vi "03122013A.vi"() -> ()   [LabVIEW 2012]
panel:
  out "Y min":dbl format="%0.2f"
  out "Y max":dbl format="%0.2f"
  in  "dt":dbl
  out "Waveform Chart 2":waveform(dbl)(graph)
  out "output waveform":waveform(dbl)
  out "XY Graph":cluster{"Y":dbl[], "Y":dbl[]}[](graph)
  out "Waveform Graph":cluster{"Xo":i32, "dx":i32, dbl[]}(graph)
  in  "Scale Legend:Visible":bool
  in  "Data on Demand":bool
  in  "X Scale.Style":u8
  out "File Status":bool
  out "Elapsed Time Text":string
  out "Waveform Chart":cluster{i32, "Elapsed Time (s)":dbl, dbl}(graph)
  in  "access (0:read/write)":enum16{"read/write", "read-only", "write-only"}(ring)
  out "output cluster":cluster{string, string, string}
  in  "operation (0:open) 2":T1(ring)
  in  "file path (use dialog) 2":path
  in  "Scan Control":dbl(knob)=250.0 scale=0.0..5000.0
  out "Data Panel":T2 {"Elapsed Time (s)" format="%#_5f"}
  out "error out":errorcluster
  out "Array":dbl[][](array[numeric])
  in  "stop":bool
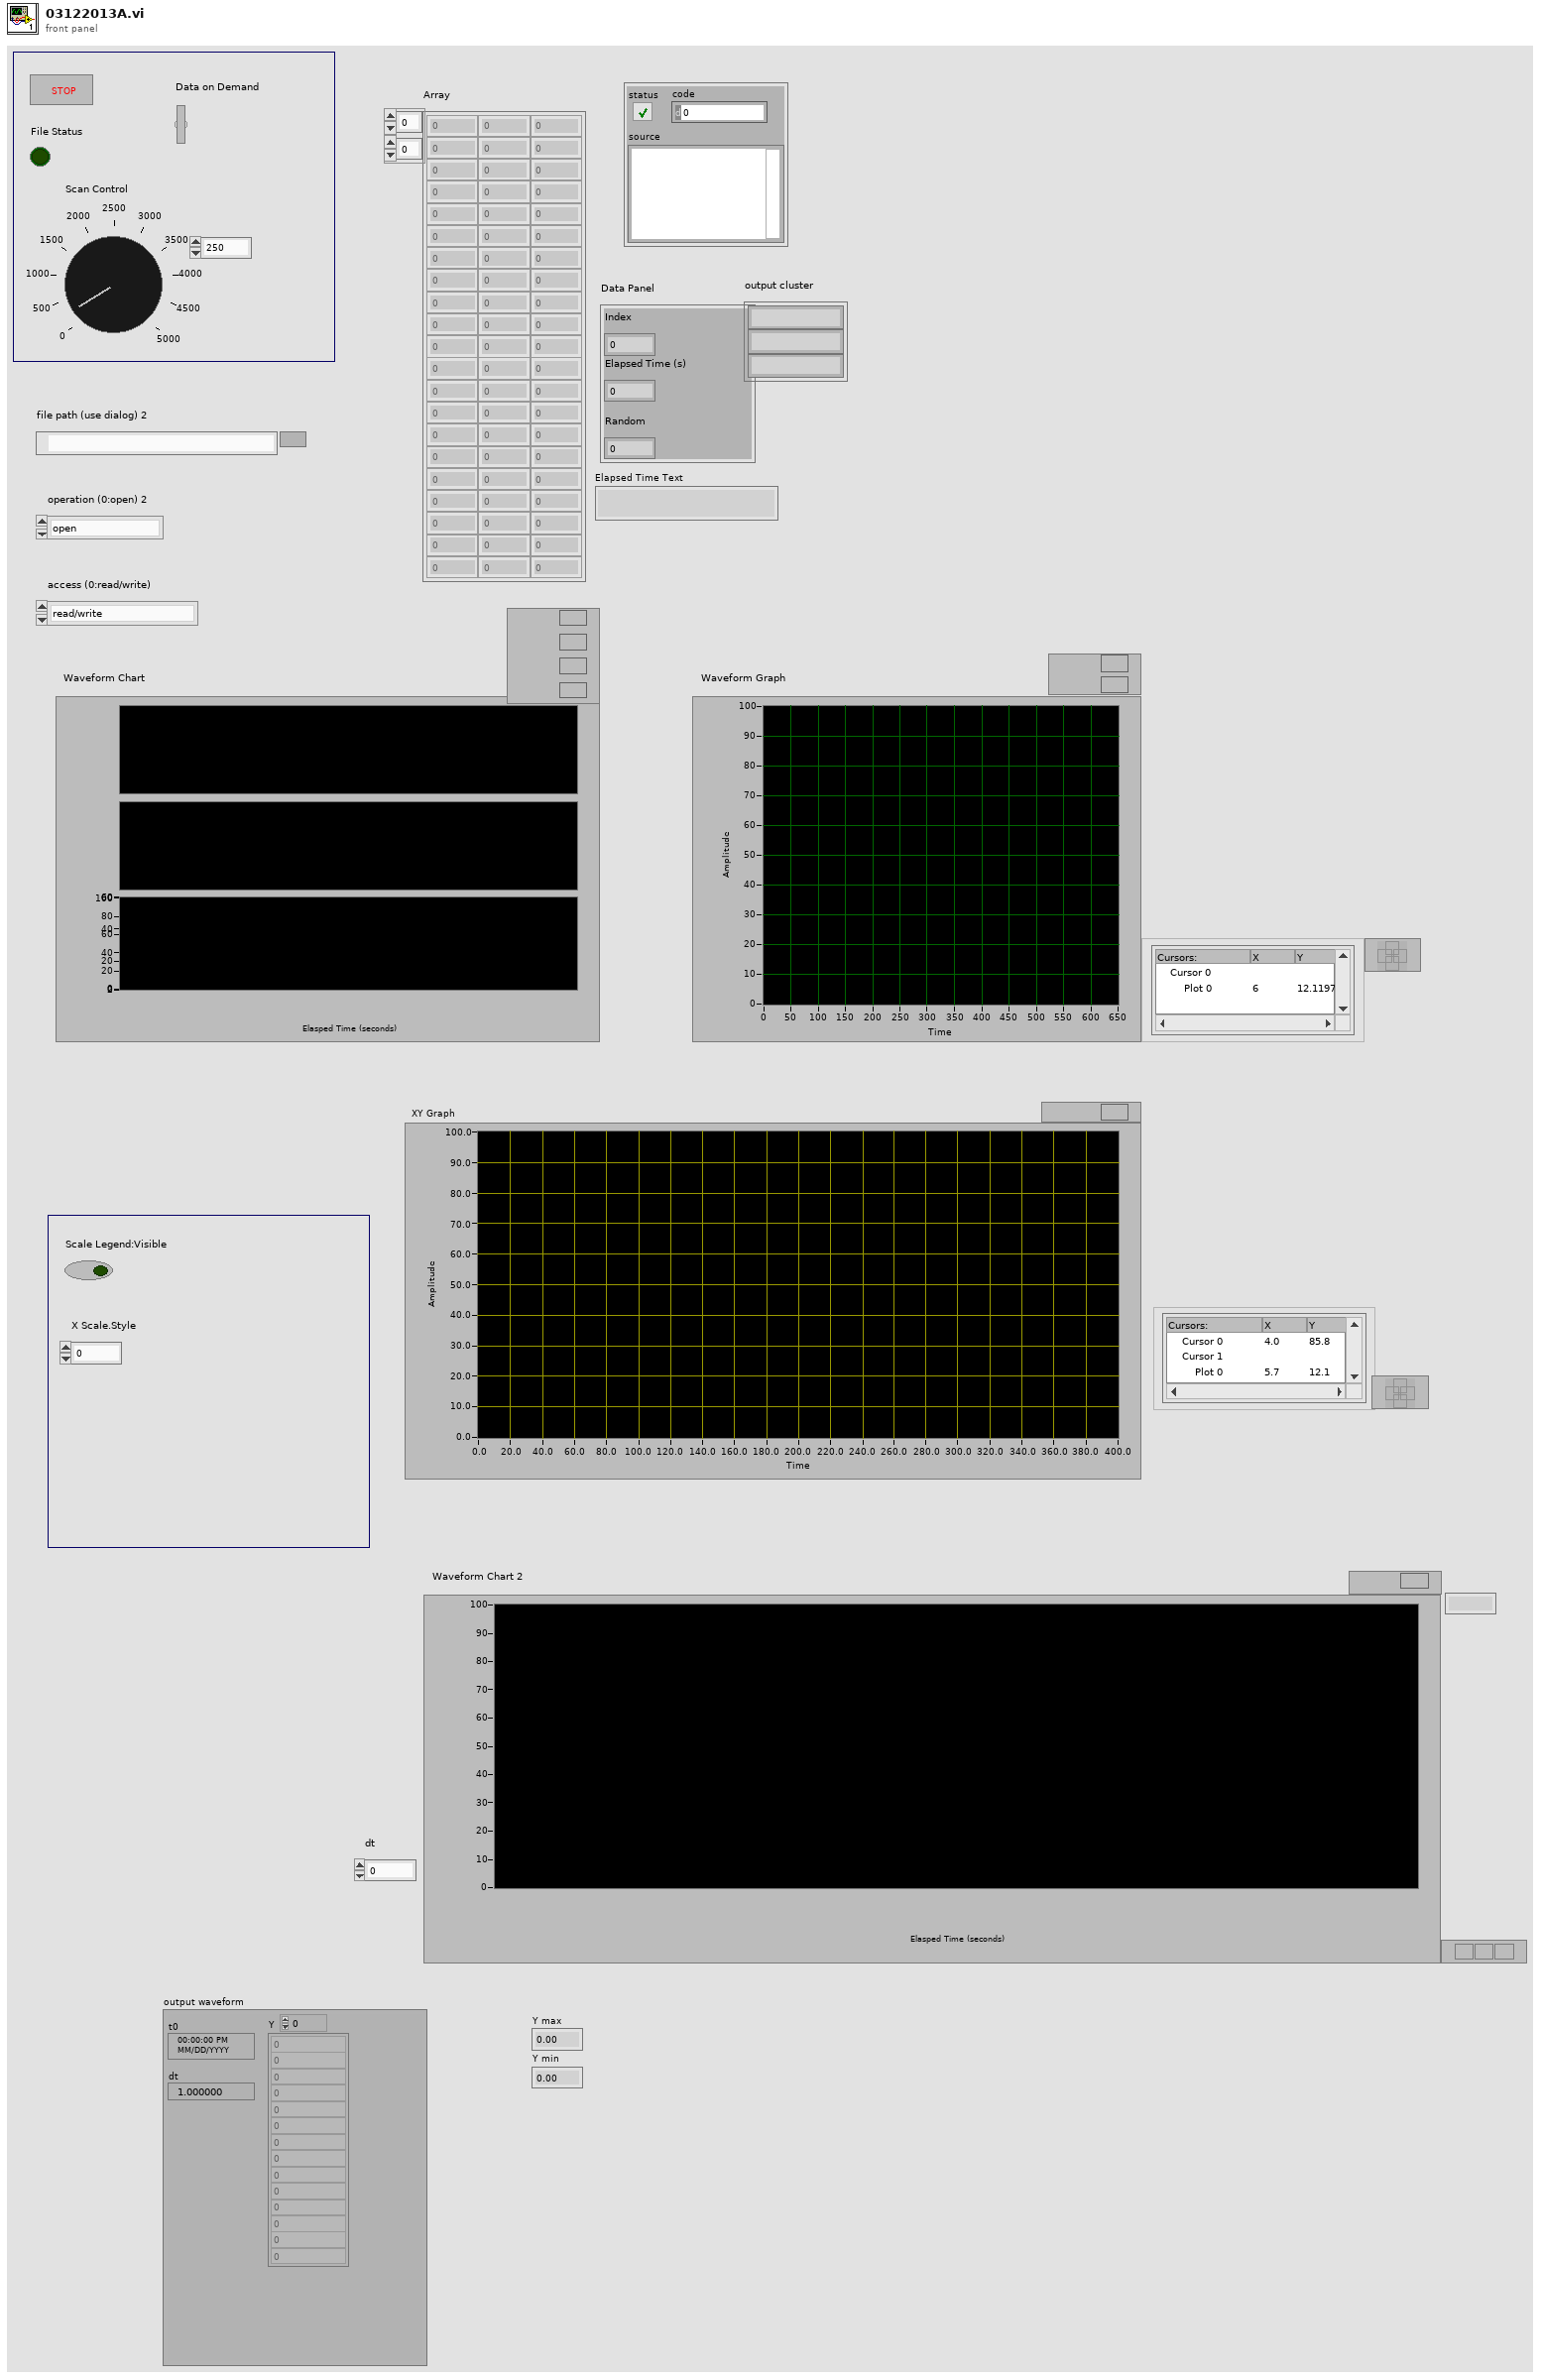
[diagram p1: front panel]
types:
  T1 = enum16{"open", "replace", "create", "open or create", "replace or create", "replace or create with confirmation"}
  T2 = cluster{"Index":i32, "Elapsed Time (s)":dbl, "Random":dbl}
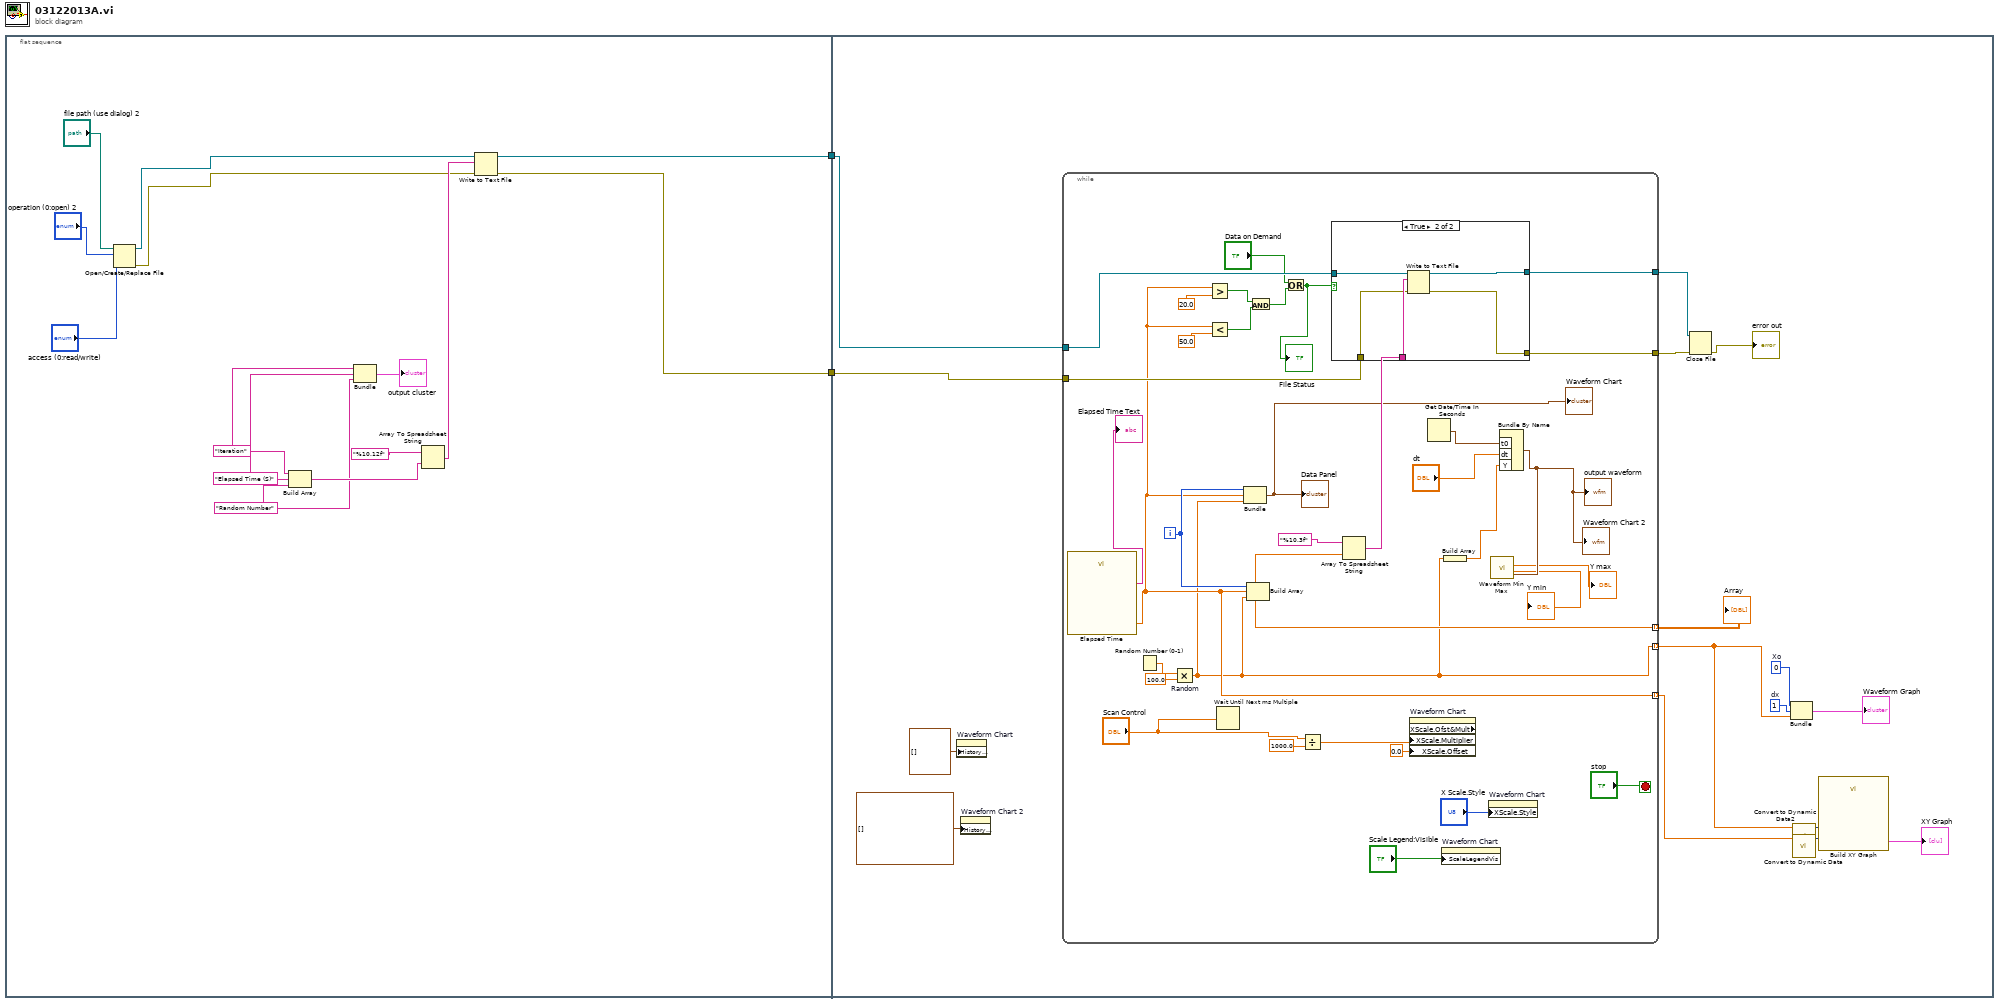
[diagram p0: block diagram]
diagram:
  n1 = flat-sequence {
    tunnel: [w4] -> w2
    tunnel: [w3] -> w1
    tunnel: w2 -> [w29]
    tunnel: w1 -> [w28]
    frame #0 {
      w8 = "Elapsed Time (S)"
      w7 = "Random Number"
      w9 = "Iteration"
      n2 = Open/Create/Replace File(file path (use dialog)="file path (use dialog) 2", operation (0:open)="operation (0:open) 2", access (0:read/write)="access (0:read/write)") -> (refnum out=w12:refnum<file>, error out=w11:errorcluster)  [unwired: 3 in, 1 out]
      n3 = Build Array(w9, w8, w7) -> (w10:string[])
      n4 = Bundle(w9, w8, w7) -> (→"output cluster":cluster{string, string, string})  [unwired: 1 in]
      n5 = Array To Spreadsheet String(array=w10, 3:"%10.12f" ("format string")) -> (spreadsheet string=w16:string)  [unwired: 1 in]
      n6 = Write to Text File(file (use dialog)=w12, text=w16, error in=w11) -> (refnum out=w4:refnum<file>, error out=w3:errorcluster)  [unwired: 1 in, 1 out]
    }
    frame #1 {
      w25 = 1  # dx
      w26 = 0  # Xo
      n7 = property on="Waveform Chart" class="WFChart (strict)"("History Data"=cluster{i32, "Elapsed Time (s)":dbl, dbl}[] []) -> ()  [unwired: 2 in, 2 out]
      n8 = property on="Waveform Chart 2" class="WFChart (strict)"("History Data"=waveform(dbl)[] []) -> ()  [unwired: 2 in, 2 out]
      n9 = while {
        tunnel: [w61] -> w31
        tunnel: [w60] -> w32
        tunnel: [w40] -> w27 mode=indexing
        tunnel: w29 -> [w58]
        tunnel: w28 -> [w57]
        tunnel: [w37] -> w20 mode=indexing
        tunnel: [w43] -> w19 mode=indexing
        i -> [w59]
        stop <- "stop" stop-if-true
        n10 = call "Elapsed Time"() -> ("Elapsed Time (s)"=w43:dbl, "Elapsed Time Text"=→"Elapsed Time Text":string)  [unwired: 12 in, 6 out]
        n11 = Random Number (0-1)() -> (number: 0 to 1=w65:dbl)
        n12 = Multiply "Random"(x=w65, y=100.0) -> (x*y=w37:dbl)
        n13 = Greater?(x=w43, y=20.0) -> (0:w53:bool)
        n14 = Less?(x=w43, y=50.0) -> (x < y?=w52:bool)
        n15 = Wait Until Next ms Multiple(millisecond multiple="Scan Control") -> ()  [unwired: 1 out]
        n16 = Bundle(w59, "Elapsed Time (s)"=w43, w37) -> (→"Data Panel" →"Waveform Chart":cluster{i32, "Elapsed Time (s)":dbl, dbl})  [unwired: 1 in]
        n17 = Build Array(w59, w43, w37) -> (w40:dbl[])
        n18 = And(x=w53, y=w52) -> (x .and. y?=w47:bool)
        n19 = Or(x="Data on Demand", y=w47) -> (x .or. y?=w46:bool)
        "File Status" <- w46
        n20 = Divide(x="Scan Control", y=1000.0) -> (x/y=w44:dbl)
        n21 = Array To Spreadsheet String(array=w40, 3:"%10.3f" ("format string")) -> (spreadsheet string=w62:string)  [unwired: 1 in]
        n22 = case shown="True" w46 {
          tunnel: w62 -> [_ w71]
          tunnel: [_ w70] -> w61
          tunnel: [_ w69] -> w60
          tunnel: w58 -> [_ w68]
          tunnel: w57 -> [_ w67]
          frame False {
          }
          frame True {
            n23 = Write to Text File(file (use dialog)=w68, text=w71, error in=w67) -> (refnum out=w69:refnum<file>, error out=w70:errorcluster)  [unwired: 1 in, 1 out]
          }
        }
        n24 = property on="Waveform Chart" class="WFChart (strict)" props=["XScale", "Ofst&Mult", "XScale", "Multiplier", "XScale", "Offset"]("XScale.Multiplier"=w44, "XScale.Offset"=0.0 ("X Scale.Offset and Multiplier:Offset")) -> ()  [unwired: 2 in, 3 out]
        n25 = Get Date/Time In Seconds() -> (seconds since 1Jan1904=w39:timestamp)
        n26 = property on="Waveform Chart" class="WFChart (strict)"("ScaleLegendVis"="Scale Legend:Visible") -> ()  [unwired: 2 in, 2 out]
        n27 = Build Array(w37) -> (w36:dbl[])
        n28 = property on="Waveform Chart" class="WFChart (strict)"("XScale.Style"="X Scale.Style") -> ()  [unwired: 2 in, 2 out]
        n29 = Bundle By Name("t0"=w39, "dt"="dt", "Y"=w36) -> (w35:waveform(dbl))  [unwired: 1 in]
        "output waveform" <- w35
        "Waveform Chart 2" <- w35
        n30 = call <vilib>:"Waveform Min Max.vi"("waveform in"=w35) -> ("Y min"=→"Y min":dbl, "Y max"=→"Y max":dbl)  [unwired: 5 in, 4 out]
      }
      "Array" <- w27
      n31 = Close File(refnum=w32, error in=w31) -> (error out=→"error out":errorcluster)  [unwired: 1 out]
      n32 = Bundle("Xo"=w26, "dx"=w25, w20) -> (→"Waveform Graph":cluster{"Xo":i32, "dx":i32, dbl[]})  [unwired: 1 in]
      n33 = call "Convert to Dynamic Data2"("Array"=w20) -> ("Dynamic Data Type"=w21:dynamicdata)  [unwired: 3 in]
      n34 = call "Convert to Dynamic Data"("Array"=w19) -> ("Dynamic Data Type"=w22:dynamicdata)  [unwired: 3 in]
      n35 = call "Build XY Graph"("Y Input"=w21, "X Input"=w22) -> ("XY Graph"=→"XY Graph":cluster{"Y":dbl[], "Y":dbl[]}[])  [unwired: 3 in, 6 out]
    }
  }
